vi "UDCPause.vi"(8 "Error In":errorcluster, 11 "Pause":bool) -> (0 "Error Out":errorcluster)   [LabVIEW 2020, in "niceiplib.lvlib"]
doc: "This API pauses the data collection as part of CEIP until unpaused. Pausing of CEIP data collection is done usually when a CPU intensive or critical operation is going on to make sure the user experience is not affected."
uses:
  <vilib>/UDC/niceiplib.lvlib
panel:
  # "@param[in]\tpause\tTrue for pausing and False for un-pausing."
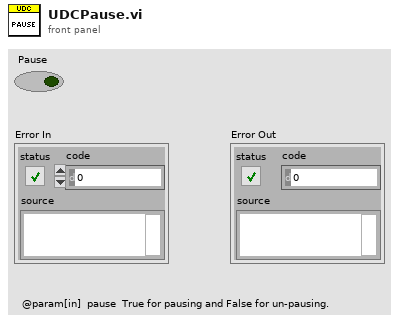
[diagram p1: front panel]
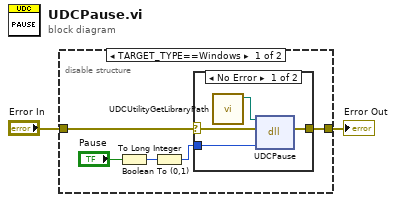
[diagram p0: block diagram]
diagram:
  n1 = disable-structure shown="TARGET_TYPE==Windows" {
    disable-tunnel: [w4 w13] -> w2
    disable-tunnel: "Error In" -> [w3 w13]
    frame condition #0 (active) {
      n2 = Boolean To (0,1)(Boolean="Pause") -> (0, 1=w6:i16)
      n3 = To Long Integer(number=w6) -> (32bit integer=w5:i32)
      n4 = case shown="No Error" w3 {
        selector: w3 -> [w9 w12]
        tunnel: w5 -> [w11 _]
        tunnel: [w10 w12] -> w4
        frame No Error {
          n5 = call <vilib>:"UDCUtilityGetLibraryPath.vi"() -> ("Library Path"=w8:path)  [unwired: 11 in]
          n6 = dll-call lib="C:/2013LabVIEWCode/dist/vi.lib/UDC/niceiplib.*" fn="UDCPause"(path in=w8, error in=w9, "pause"=w11) -> (error out=w10:errorcluster)  [unwired: 3 in, 1 out]
        }
        frame Error {
        }
      }
    }
    frame condition #1 {
    }
  }
  "Error Out" <- w2
